vi "Start Module.vi"(7 "Panel":refnum<class "Panel.lvclass"> caption="Panel (Window)", 8 "error in (no error)":errorcluster) -> (0 "error out":errorcluster, 1 "Wait for Event Sync?":bool, 2 "Data Logger v2 Broadcast Events":T1, 3 "Module Was Already Running?":bool)   [LabVIEW 2025, in "Data Logger v2.lvlib"]
doc: "Launches the Module Main.vi.\n_____\nBased on Delacor QMH Project Template 3.1.0.34."
uses:
  Data Logger v2.lvlib
  Broadcast Events--cluster.ctl
  Did Init Argument--cluster.ctl
  Status Updated Argument--cluster.ctl
  Error Reported Argument--cluster.ctl
  Stop Argument--cluster.ctl
  Get Module Execution Status Argument--cluster.ctl
  <vilib>/MGI/Panel Manager/Panel/Panel/Panel.lvclass
  <vilib>/Delacor/Delacor QMH/Libraries/Module Admin_class/Delacor_lib_QMH_Module Admin.lvclass
  <vilib>/Delacor/Delacor QMH/Libraries/Module Admin_class/Delacor_lib_QMH_Module Admin.lvclass/Delacor_lib_QMH_Module Admin.ctl
  <vilib>/Delacor/Delacor QMH/Libraries/Module Admin_class/Delacor_lib_QMH_Set External Launch.vi
  <vilib>/MGI/Panel Manager/Panel/Panel/Window/Window.lvclass
  C:/Program Files/National Instruments/LabVIEW 2025/vi.lib/MGI/Panel Manager/Panel/Panel/Panel.lvclass
  <vilib>/MGI/Panel Manager/Panel/Panel/Window/Window.vi
  <vilib>/Utility/error.llb/Error Cluster From Error Code.vi
  <vilib>/ErrorRing/Error Ring.xnode
  <vilib>/MGI/Panel Manager/Panel/Panel.lvlib
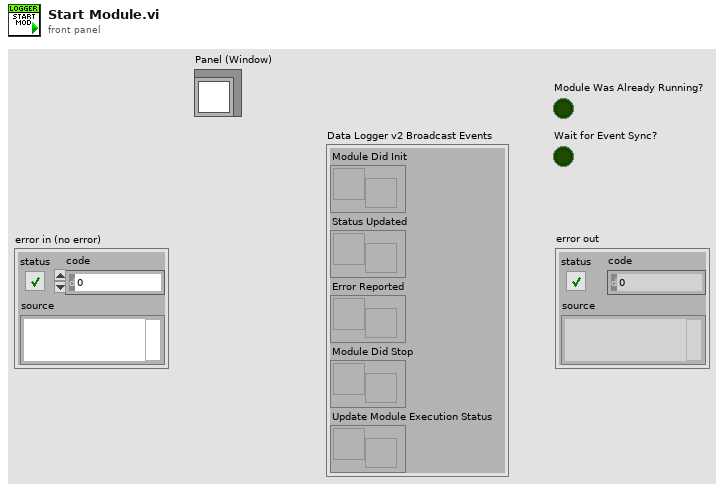
[diagram p1: front panel]
types:
  T1 = typedef "Data Logger v2.lvlib/Broadcast Events--cluster.ctl" = cluster{"Module Did Init":refnum<user-event>, "Status Updated":refnum<user-event>, "Error Reported":refnum<user-event>, "Module Did Stop":refnum<user-event>, "Update Module Execution Status":refnum<user-event>}
  T2 = enum32{"Bad", "Idle", "Run top level", "Running"}
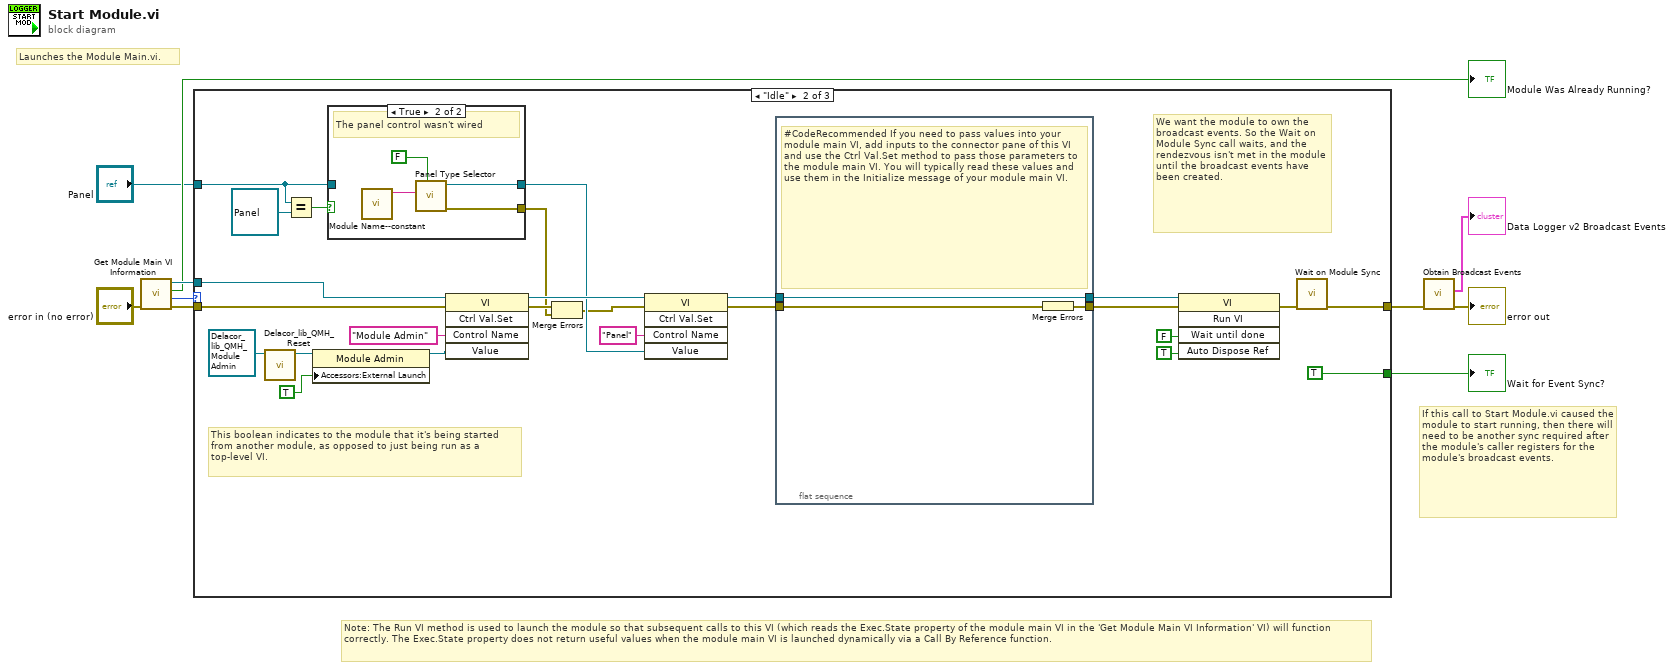
[diagram p0: block diagram]
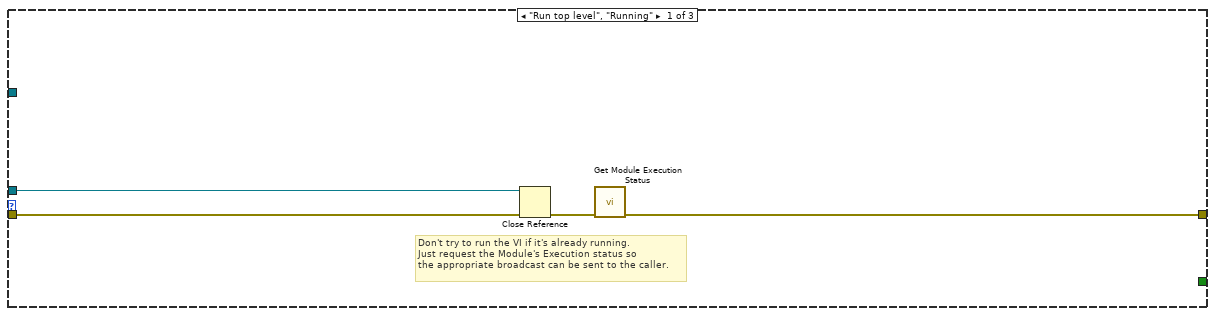
[diagram p2: hidden frame]
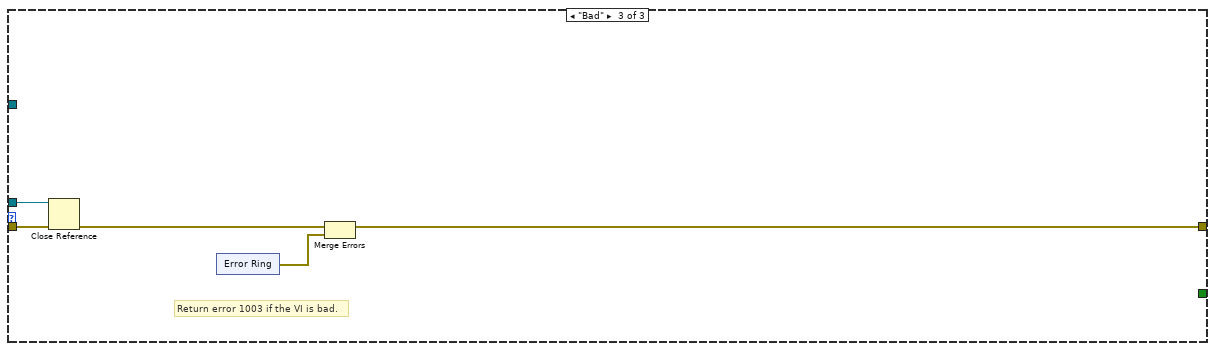
[diagram p4: hidden frame]
diagram:
  # "Note: The Run VI method is used to launch the module so that subsequent calls to this VI (which reads the Exec.State property of the module main VI in the 'Get Module Main VI Information' VI) will function correctly. The Exec.State property does not return useful values when the module main VI is launched dynamically via a Call By Reference function."
  # "If this call to Start Module.vi caused the module to start running, then there will need to be another sync required after the module's caller registers for the module's broadcast events."
  # "Launches the Module Main.vi."
  n1 = call "Get Module Main VI Information.vi"("error in (no error)"="error in (no error)") -> ("error out"=w9:errorcluster, "Execution State"=w4:T2, "Is Module Running?"=→"Module Was Already Running?":bool, "Module Main VI"=w8:refnum<vi>)  [unwired: 7 in]
  n2 = case shown="\"Idle\"" w4 {
    tunnel: w9 -> [w14 w37 w52]
    tunnel: w8 -> [w13 w38 w51]
    tunnel: [w11 w21 w49] -> w7
    tunnel: [_ TRUE _] -> w5
    tunnel: "Panel" -> [_ w18 _]
    frame "Run top level", "Running" {
      # "Don't try to run the VI if it's already running.\nJust request the Module's Execution status so\nthe appropriate broadcast can be sent to the caller."
      n3 = Close Reference(reference=w13, error in (no error)=w14) -> (error out=w12:errorcluster)
      n4 = call "Get Module Execution Status.vi"("error in (no error)"=w12) -> ("error out"=w11:errorcluster)  [unwired: 10 in]
    }
    frame "Idle" {
      # "We want the module to own the broadcast events. So the Wait on Module Sync call waits, and the rendezvous isn't met in the module until the broadcast events have been created."
      # "This boolean indicates to the module that it's being started from another module, as opposed to just being run as a top-level VI."
      n5 = call-dynamic "Delacor_lib_QMH_Reset.vi"("Mod Admin in"=refnum<class "Delacor_lib_QMH_Module Admin.lvclass"> refnum) -> ("Mod Admin out"=w33:refnum<class "Delacor_lib_QMH_Module Admin.lvclass">)  [unwired: 9 in, 1 out]
      n6 = Equal?(x=w18, y=refnum<class "Panel.lvclass"> refnum) -> (x = y?=w19:bool)
      n7 = property class="Module Admin"(reference=w33, "Accessors:External Launch"=TRUE) -> (reference out=w30:refnum<class "Delacor_lib_QMH_Module Admin.lvclass">)  [unwired: 1 in, 1 out]
      n8 = case shown="True" w19 {
        tunnel: w18 -> [w40 _]
        tunnel: [w40 w44] -> w17
        tunnel: [_ w41] -> w15
        frame False {
          # "A panel object was wired in."
        }
        frame True {
          # "The panel control wasn't wired"
          n9 = call "Module Name--constant.vi"() -> ("Module Name"=w42:string)  [unwired: 11 in]
          n10 = call-poly <vilib>:"Panel Type Selector.vi"("Autoshow? (T)"=FALSE, "Default Title"=w42) -> ("error out"=w41:errorcluster, "Window out"=w44:refnum<class "Window.lvclass">)  [unwired: 8 in]
        }
      }
      n11 = invoke class="VI" method="Ctrl Val.Set"(reference=w38, error in=w37, "Control Name"="Module Admin", "Value"=w30) -> (reference out=w26:refnum<vi>, error out=w25:errorcluster)  [unwired: 1 in, 3 out]
      n12 = Merge Errors(w25, w15) -> (w16:errorcluster)
      n13 = invoke class="VI" method="Ctrl Val.Set"(reference=w26, error in=w16, "Control Name"="Panel", "Value"=w17) -> (reference out=w24:refnum<vi>, error out=w23:errorcluster)  [unwired: 1 in, 3 out]
      n14 = flat-sequence {
        tunnel: w24 -> [w47]
        tunnel: [w47] -> w29
        tunnel: w23 -> [w46]
        tunnel: [w45] -> w28
        frame #0 {
          # "#CodeRecommended If you need to pass values into your module main VI, add inputs to the connector pane of this VI and use the Ctrl Val.Set method to pass those parameters to the module main VI. You will typically read these values and use them in the Initialize message of your module main VI."
          n15 = Merge Errors(w46) -> (w45:errorcluster)
        }
      }
      n16 = invoke class="VI" method="Run VI"(reference=w29, error in=w28, "Wait until done"=FALSE ("Wait Until Done"), "Auto Dispose Ref"=TRUE ("Auto Dispose Reference")) -> (error out=w22:errorcluster)  [unwired: 1 in, 4 out]
      n17 = call "Wait on Module Sync.vi"("error in (no error)"=w22) -> ("error out"=w21:errorcluster)  [unwired: 10 in]
    }
    frame "Bad" {
      # "Return error 1003 if the VI is bad."
      n18 = Close Reference(reference=w51, error in (no error)=w52) -> (error out=w50:errorcluster)
      n19 = xnode "Error Ring"() -> ("error out"=w48:errorcluster)
      n20 = Merge Errors(w50, w48) -> (w49:errorcluster)
    }
  }
  "Wait for Event Sync?" <- w5
  n21 = call "Obtain Broadcast Events.vi"("error in (no error)"=w7) -> ("error out"=→"error out":errorcluster, "Data Logger v2 Broadcast Events"=→"Data Logger v2 Broadcast Events":T1)  [unwired: 9 in]
